vi "Evaluate Stop Trigger.vi"(1 "Enable":bool, 2 "Stop Trigger":bool) -> (7 "Stop current grab":bool)   [LabVIEW 2014]
panel:
  # "Copyright 2014 Vidrio Technologies\nScanImage 5 software is licensed under the Apache License, Version 2.0 (the \"License\"); you may not use any files contained\nwithin the ScanImage 5 release except in compliance with the License. You may obtain a copy of the License at\n http://www.apache.org/licenses/LICENSE-2.0\nUnless required by applicable law or agreed to in writing, software distributed under the License is distributed on an\n\"AS IS\" BASIS, WITHOUT WARRANTIES OR CONDITIONS OF ANY KIND, either express or implied. See the License for the\n specific language governing permissions and limitations under the License."
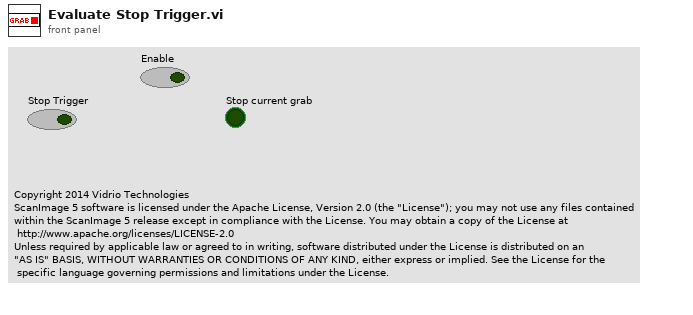
[diagram p1: front panel]
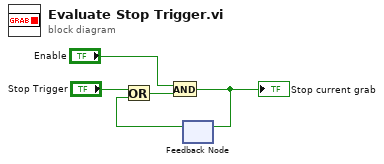
[diagram p0: block diagram]
diagram:
  n1 = feedback #1() -> (w5:bool)  [unwired: 1 in]
  n2 = Or(x="Stop Trigger", y=w5) -> (x .or. y?=w4:bool)
  n3 = And(x="Enable", y=w4) -> (x .and. y?=w3:bool)
  "Stop current grab" <- w3
  n4 = feedback-in #1(w3) -> ()
